vi "Get Enum Type Specializations.vi"(8 "error in (no error)":errorcluster, 10 "measurement control path":path, 11 "MeasurementPluginService in":refnum<class "MeasurementPluginService.lvclass">) -> (0 "error out":errorcluster, 2 "Type Specializations":T1[](array[typedef]), 3 "MeasurementPluginService out":refnum<class "MeasurementPluginService.lvclass">)   [LabVIEW 2020, in "MeasurementLink Measurement Server.lvlib"]
uses:
  MeasurementLink Measurement Server.lvlib
  Classes/MeasurementPluginService/MeasurementPluginService.lvclass
  TypeDefs/Parameter Type Specialization.ctl
  TypeDefs/Type Specialization.ctl
  TypeDefs/Type Specialization Key.ctl
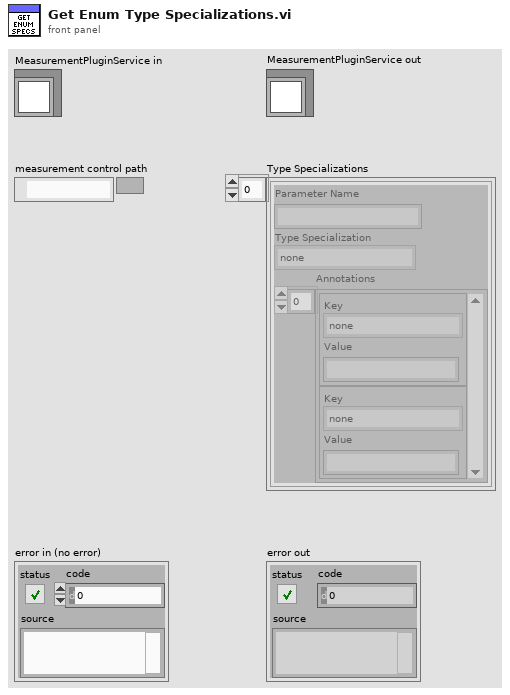
[diagram p1: front panel]
types:
  T1 = typedef "MeasurementLink Measurement Server.lvlib/Parameter Type Specialization.ctl" = cluster{"Parameter Name":string, "Type Specialization":T2, "Annotations":cluster{"Key":T3, "Value":string}[]}
  T2 = typedef "MeasurementLink Measurement Server.lvlib/Type Specialization.ctl" = enum16{"none", "pin", "path", "enum"}
  T3 = typedef "MeasurementLink Measurement Server.lvlib/Type Specialization Key.ctl" = enum16{"none", "pin.instrument_type", "enum.values"}
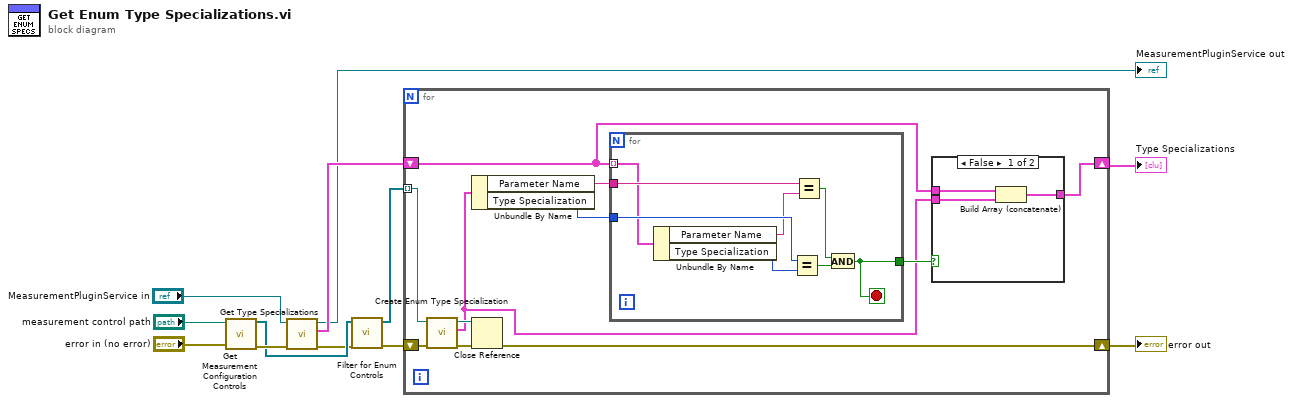
[diagram p0: block diagram]
diagram:
  n1 = call "Get Measurement Configuration Controls.vi"("error in (no error)"="error in (no error)", "measurement configuration control path"="measurement control path") -> ("error out"=w11:errorcluster, "Controls[]"=w9:refnum<vi>[])  [unwired: 7 in]
  n2 = call-dynamic "Get Type Specializations.vi"("error in (no error)"=w11, "MeasurementPluginService in"="MeasurementPluginService in") -> ("error out"=w8:errorcluster, "Type Specializations"=w12:T1[], "MeasurementPluginService out"=→"MeasurementPluginService out":refnum<class "MeasurementPluginService.lvclass">)  [unwired: 7 in]
  n3 = call "Filter for Enum Controls.vi"("error in (no error)"=w8, "Controls[]"=w9) -> ("error out"=w10:errorcluster, "Enum Controls[]"=w7:refnum<vi>[])  [unwired: 8 in]
  n4 = for {
    shift-right: [w18] -> w5
    shift-left: w10 -> [w14]
    tunnel: w7 -> [w13] mode=indexing
    shift-right: [w15] -> w6
    shift-left: w12 -> [w16]
    n5 = call "Create Enum Type Specialization.vi"("error in (no error)"=w14, "Enum reference in"=w13) -> ("error out"=w20:errorcluster, "Parameter Type Specialization Output"=w17:T1, "Control reference out"=w19:refnum<vi>)  [unwired: 6 in]
    n6 = Unbundle By Name(w17) -> ("Parameter Name"=w23:string, "Type Specialization"=w22:T2)
    n7 = Close Reference(reference=w19, error in (no error)=w20) -> (error out=w18:errorcluster)
    n8 = for {
      tunnel: w23 -> [w33]
      tunnel: w22 -> [w34]
      tunnel: [w29] -> w21
      tunnel: w16 -> [w28] mode=indexing
      stop <- w29 stop-if-true
      n9 = Unbundle By Name(w28) -> ("Parameter Name"=w32:string, "Type Specialization"=w35:T2)
      n10 = Equal?(x=w34, y=w35) -> (x = y?=w30:bool)
      n11 = Equal?(x=w33, y=w32) -> (x = y?=w31:bool)
      n12 = And(x=w31, y=w30) -> (x .and. y?=w29:bool)
    }
    n13 = case shown="False" w21 {
      tunnel: w16 -> [w26 w27]
      tunnel: w17 -> [w24 _]
      tunnel: [w25 w27] -> w15
      frame False {
        n14 = Build Array (concatenate)(w26, w24) -> (w25:T1[])
      }
      frame True {
      }
    }
  }
  "Type Specializations" <- w6
  "error out" <- w5
